vi "testString Comparison.vi"(8 "error in (no error)":errorcluster, 11 "TestCase in":refnum<class "VITAC Example Test Case.lvclass">) -> (0 "error out":errorcluster, 3 "TestCase out":refnum<class "VITAC Example Test Case.lvclass">)   [LabVIEW 2015, in "VITAC Example Test Case.lvclass"]
uses:
  VITAC Example Test Case.lvclass
  <vilib>/addons/_JKI Toolkits/VI Tester/TestCase.llb/TestCase.lvclass
  <vilib>/Wiresmith Technology/VITAC (VI Tester Advanced Comparisons)/VITAC.lvlib
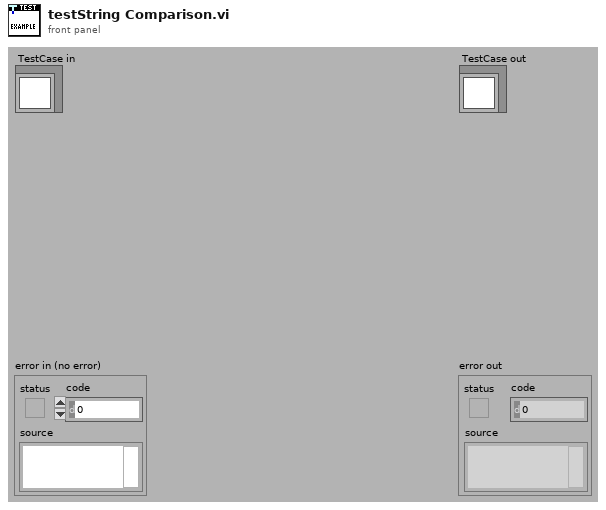
[diagram p1: front panel]
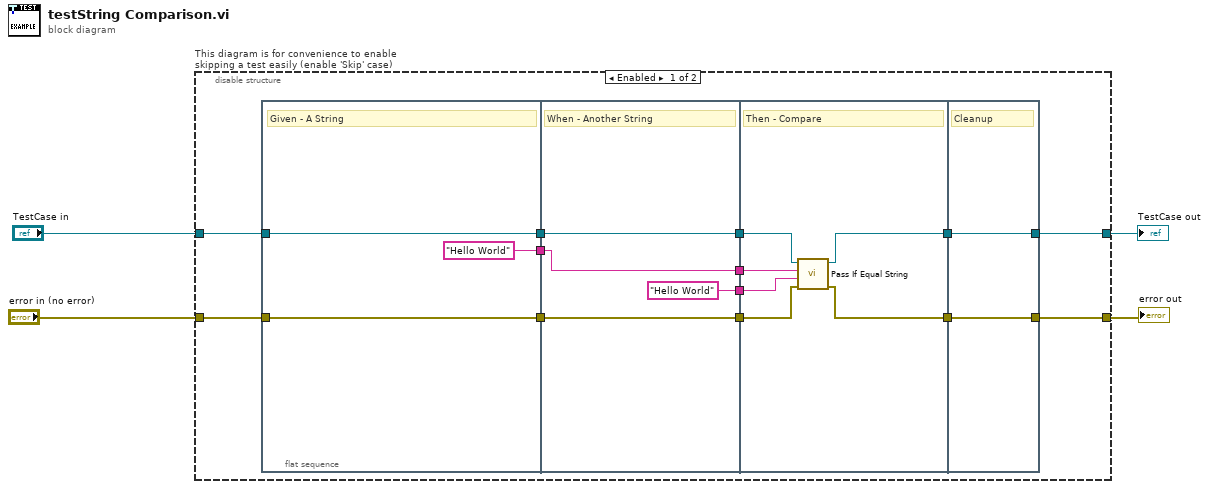
[diagram p0: block diagram]
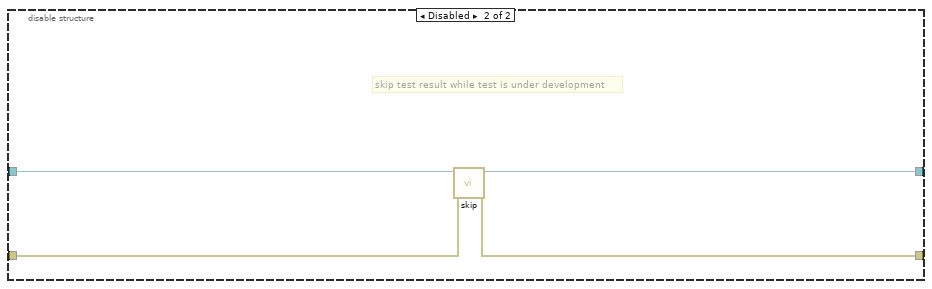
[diagram p2: hidden frame]
diagram:
  n1 = disable-structure "This diagram is for convenience to enable skipping a test easily (enable 'Skip' case)" shown="Enabled" {
    disable-tunnel: "TestCase in" -> [w11 w36]
    disable-tunnel: [w9 w34] -> w1
    disable-tunnel: [w8 w35] -> w3
    disable-tunnel: "error in (no error)" -> [w10 w33]
    frame Enabled {
      n2 = flat-sequence {
        tunnel: w10 -> [w19]
        tunnel: w11 -> [w20]
        tunnel: [w20] -> w17
        tunnel: [w19] -> w16
        tunnel: ["Hello World"] -> w7
        tunnel: [w24] -> w15
        tunnel: [w23] -> w14
        tunnel: w17 -> [w24]
        tunnel: w16 -> [w23]
        tunnel: w7 -> [w22]
        tunnel: [w22] -> w6
        tunnel: ["Hello World"] -> w5
        tunnel: [w29] -> w13
        tunnel: [w27] -> w12
        tunnel: w15 -> [w30]
        tunnel: w14 -> [w28]
        tunnel: w6 -> [w26]
        tunnel: w5 -> [w25]
        tunnel: [w31] -> w8
        tunnel: [w32] -> w9
        tunnel: w13 -> [w32]
        tunnel: w12 -> [w31]
        frame #0 {
          # "Given - A String"
        }
        frame #1 {
          # "When - Another String"
        }
        frame #2 {
          # "Then - Compare"
          n3 = call <vilib>:"Pass If Equal String.vi"("error in (no error)"=w28, "actual"=w25, "expected"=w26, "TestCase in"=w30) -> ("error out"=w27:errorcluster, "TestCase out"=w29:refnum<class "VITAC Example Test Case.lvclass">)  [unwired: 6 in]
        }
        frame #3 {
          # "Cleanup"
        }
      }
    }
    frame Disabled {
      # "skip test result while test is under development"
      n4 = call <vilib>:"skip.vi"("error in (no error)"=w33, "TestCase in"=w36) -> ("error out"=w35:errorcluster, "TestCase out"=w34:refnum<class "VITAC Example Test Case.lvclass">)  [unwired: 8 in]
    }
  }
  "error out" <- w3
  "TestCase out" <- w1
